vi "Command Loop - Get HW Values.vi"(8 "error in":errorcluster, 10 "Data":string, 11 "Queue Refs in":variant) -> (0 "error out":errorcluster, 2 "Response":string, 3 "Queue Refs out":variant)   [LabVIEW 2026, in "Runtime Configuration Support Example Engine.lvlib"]
uses:
  Runtime Configuration Support Example Engine.lvlib
  <vilib>/NI VeriStand/Custom Device API/Custom Device Item Ref.ctl
  <vilib>/NI VeriStand/Custom Device API/Custom Device API.lvlib
  Shared/Compiled.Settings.ctl
  Shared/Runtime Configuration Support Example Shared.lvlib
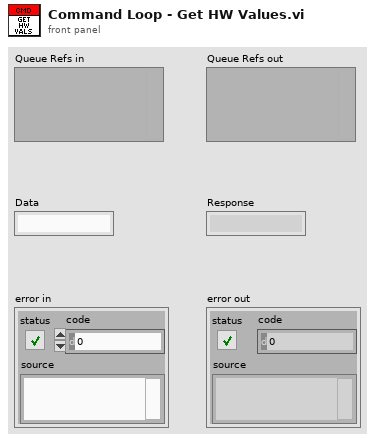
[diagram p1: front panel]
types:
  T1 = cluster{"Compiled Info":refnum<queue>, "Set HW Val Ref":refnum<queue>, "Get HW Val Ref":refnum<queue>}
  T2 = cluster{"In Indices":i32[], "Out Indices":i32[], "In Values":i32[], "Out Values":i32[], "Error":errorcluster}
  T3 = cluster{"SignalIDs In":i32[], "SignalIDs Out":i32[], "Response Ref":refnum<queue>}
  T4 = cluster{"SignalIDsIn":i32[], "SignalIDsOut":i32[]}
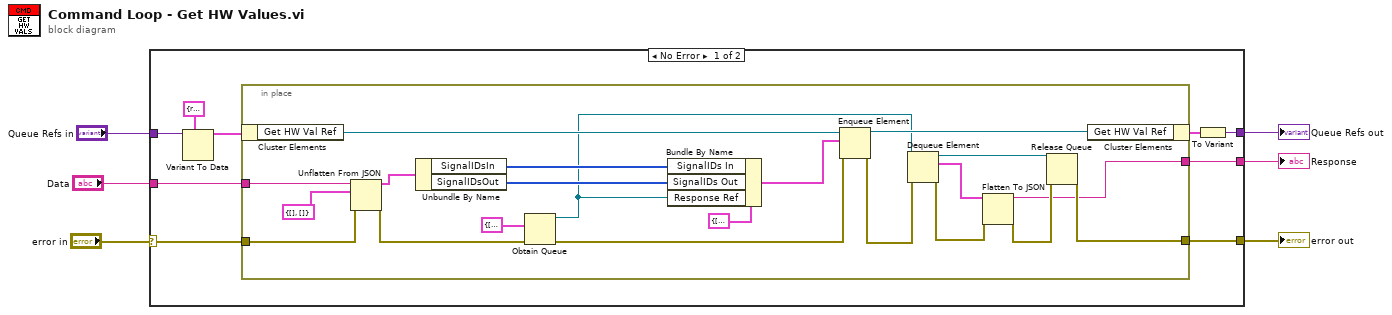
[diagram p0: block diagram]
diagram:
  n1 = case shown="No Error" "error in" {
    selector: "error in" -> [w15 w38]
    tunnel: "Data" -> [w13 _]
    tunnel: "Queue Refs in" -> [w11 w37]
    tunnel: [w14 w38] -> w5
    tunnel: [w12 _] -> w3
    tunnel: [w8 w37] -> w1
    frame No Error {
      n2 = Variant To Data(type=T1 {"Compiled Info"=refnum, "Set HW Val Ref"=refnum, "Get HW Val Ref"=refnum} ("Queue Refs in"), Variant=w11) -> (data=w10:T1)  [unwired: 1 in, 1 out]
      n3 = in-place {
        in-place-border: w15 -> [w36]
        in-place-border: [w34] -> w14
        in-place-border: w13 -> [w17]
        in-place-border: [w26] -> w12
        n4 = in-place-cluster #1(w10) -> ("Get HW Val Ref"=w28:refnum<queue>)
        n5 = Unflatten From JSON(JSON string=w17, type and defaults=T4 {"SignalIDsIn"=[], "SignalIDsOut"=[]} ("Cluster"), error in (no error)=w36) -> (value=w22:T4, error out=w31:errorcluster)  [unwired: 4 in]
        n6 = Unbundle By Name(w22) -> ("SignalIDsIn"=w21:i32[], "SignalIDsOut"=w20:i32[])
        n7 = Obtain Queue(element data type=T2 {"In Indices"=[], "Out Indices"=[], "In Values"=[], "Out Values"=[], "Error"={"status"=FALSE, "code"=0, "source"=""}}, error in (no error)=w31) -> (queue out=w16:refnum<queue>, error out=w32:errorcluster)  [unwired: 3 in, 1 out]
        n8 = Bundle By Name(cluster=T3 {"SignalIDs In"=[], "SignalIDs Out"=[], "Response Ref"=refnum}, "SignalIDs In"=w21, "SignalIDs Out"=w20, "Response Ref"=w16) -> (w18:T3)
        n9 = Enqueue Element(queue=w28, element=w18, error in (no error)=w32) -> (queue out=w27:refnum<queue>, error out=w30:errorcluster)  [unwired: 1 in, 1 out]
        n10 = Dequeue Element(queue=w16, error in (no error)=w30) -> (queue out=w25:refnum<queue>, element=w29:T2, error out=w33:errorcluster)  [unwired: 1 in, 1 out]
        n11 = Flatten To JSON(anything=w29, error in (no error)=w33) -> (JSON string=w26:string, 11:w35:errorcluster)  [unwired: 1 in]
        n12 = Release Queue(queue=w25, error in (no error)=w35) -> (error out=w34:errorcluster)  [unwired: 1 in, 2 out]
        n13 = in-place-cluster #1("Get HW Val Ref"=w27) -> (w7:T1)
      }
      n14 = To Variant(anything=w7) -> (Variant=w8:variant)
    }
    frame Error {
    }
  }
  "error out" <- w5
  "Response" <- w3
  "Queue Refs out" <- w1
